vi "E700-Frequency Setting.vi"(8 "error in (no error)":errorcluster, 11 "Frequencey Setting (Hz)":dbl) -> (0 "error out":errorcluster, 3 "Set Value":u16)   [LabVIEW 2020]
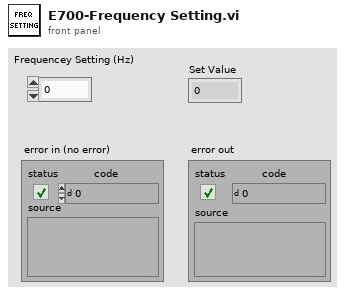
[diagram p1: front panel]
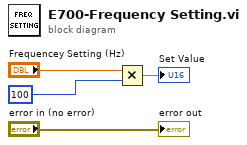
[diagram p0: block diagram]
diagram:
  n1 = Multiply(x="Frequencey Setting (Hz)", y=u16 100) -> (x*y=→"Set Value":dbl)
  "error out" <- "error in (no error)"
